vi "Stop Core.vi"(10 "final error code":i32, 11 "Connection Handler in":refnum<class "Connection Handler.lvclass">) -> (3 "Connection Handler out":refnum<class "Connection Handler.lvclass">)   [LabVIEW 2017, in "Connection Handler.lvlib" / "Connection Handler.lvclass"]
doc: "(<B>Filename</B>: Actor Framework.lvlib:Actor.lvclass:Stop Core.vi)\n\nDefines what the actor does before it stops. Use the <B>final error code</B> input to determine whether the actor shut down in response to an error.\n\nBy default, this method does nothing. A descendant class may override it to define behavior, such as shutting down any processes the actor initiated in its override of the Actor Core method."
uses:
  Connection Handler.lvclass
  Applications/National Instruments/LabVIEW 2017 64-bit/vi.lib/ActorFramework/Actor/Actor.lvclass
  <vilib>/ActorFramework/Actor/Actor.lvclass/Actor.ctl
  Connection Handler.lvclass/Connection Handler.ctl
  Connection Listener/Connection Listener Messages/Remove Connection Msg/Remove Connection Msg.lvclass/Remove Connection Msg.ctl
  <vilib>/ActorFramework/Message Enqueuer/Message Enqueuer.lvclass/Message Enqueuer.ctl
  <vilib>/ActorFramework/Message Enqueuer/Enqueue.vi
  Connection Listener/Connection Listener Messages/Remove Connection Msg/Remove Connection Msg.lvclass
  Applications/National Instruments/LabVIEW 2017 64-bit/vi.lib/ActorFramework/Message/Message.lvclass
  <vilib>/ActorFramework/Message Priority Queue/Priority Enqueue.vi
  Actor wHelper/Actor wHelper/Actor wHelper.lvclass
  <vilib>/MediaMongrels Ltd/WebSockets/Sockets/Socket/Socket.lvclass
  <vilib>/ActorFramework/Actor/Actor.lvclass
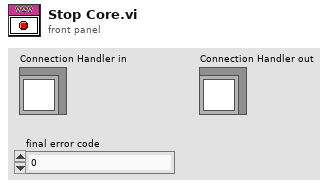
[diagram p1: front panel]
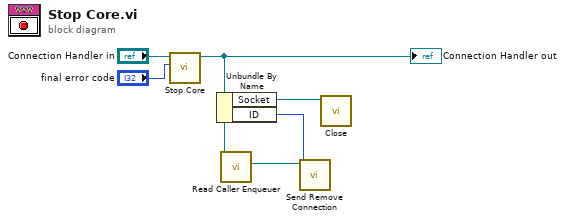
[diagram p0: block diagram]
diagram:
  n1 = call-parent "Stop Core.vi"("final error code"="final error code", "Actor wHelper in"="Connection Handler in") -> ("Actor wHelper out"=w3:refnum<class "Connection Handler.lvclass">)  [unwired: 9 in]
  "Connection Handler out" <- w3
  n2 = Unbundle By Name(w3) -> ("Socket"=w4:refnum<class "Socket.lvclass">, "ID"=w1:i32)
  n3 = call <vilib>:"Read Caller Enqueuer.vi"("Actor"=w3) -> ("Caller Enqueuer"=w2:refnum<class "Message Enqueuer.lvclass">)  [unwired: 10 in]
  n4 = call "Send Remove Connection.vi"("ID"=w1, "Message Enqueuer in"=w2) -> ()  [unwired: 8 in, 2 out]
  n5 = call-dynamic "Close.vi"("Socket in"=w4) -> ()  [unwired: 10 in, 1 out]
